vi "Get Server.vi"(8 "error in (no error)":errorcluster, 10 "id":i32, 11 "Variant in":variant) -> (0 "error out":errorcluster, 3 "Data Value Reference out":refnum<data-value>)   [LabVIEW 2020, in "MCP Server.lvlib"]
doc: "Reads one Server from the variant lookup table."
uses:
  MCP Server.lvlib
  Server Data.ctl
  Tool Data.ctl
  Input Parameter.ctl
  Output Parameter.ctl
  Logging.ctl
  User Events.ctl
  onRpc.ctl
  Prompt Data.ctl
  Prompt Argument.ctl
  resource data.ctl
  <vilib>/IlluminatedG/IG HTTP Server/HTTP Server/server/Server.lvclass
  <vilib>/Utility/error.llb/Error Cluster From Error Code.vi
  <vilib>/ErrorRing/Error Ring.xnode
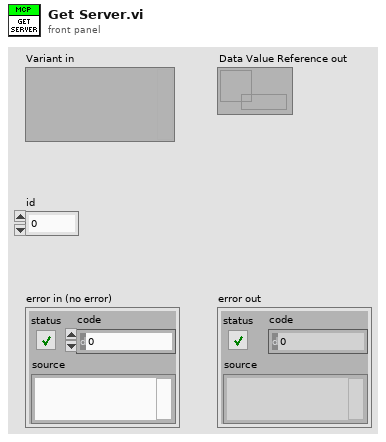
[diagram p1: front panel]
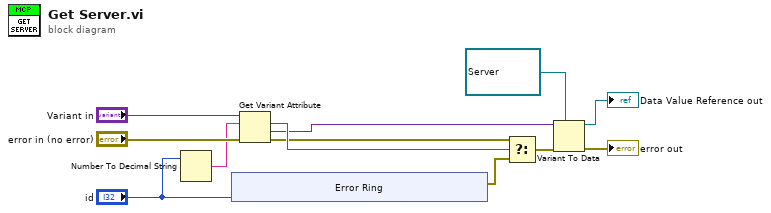
[diagram p0: block diagram]
diagram:
  n1 = Number To Decimal String(number="id") -> (decimal integer string=w1:string)  [unwired: 1 in]
  n2 = xnode "Error Ring"("parameter 0"="id") -> ("error out"=w9:errorcluster)
  n3 = Get Variant Attribute(Variant="Variant in", name=w1, error in="error in (no error)") -> (found=w8:bool, value=w5:variant, error out=w2:errorcluster)  [unwired: 1 in, 1 out]
  n4 = Select(t=w2, s=w8, f=w9) -> (s? t:f=w7:errorcluster)
  n5 = Variant To Data(error in=w7, type=refnum<data-value> refnum ("data value reference"), Variant=w5) -> (data=→"Data Value Reference out":refnum<data-value>, error out=→"error out":errorcluster)
